vi "OAT Polar Plot Cursor Name on Picture.vi"(4 "avoid rect":T1(array[cluster]), 5 "[user-specified font]":T3, 6 "name above cursor":i32=5, 7 "desired font(Application)":T4(ring)=enum."Application Font", 8 "name":string, 9 "cursor position":cluster{"horizontal":i16, "vertical":i16}, 10 "cursor attributes":T5={"layout color"=852223, "active color"=16740820, "precision"=2, "BG transparent? (T)"=FALSE, "radius"=2}, 11 "picture":picture) -> (0 "text plotted":bool, 1 "text rect":T2, 3 "new picture":picture)   [LabVIEW 2017]
uses:
  <vilib>/addons/Sound and Vibration/Order Analysis/Backward Compatibility/SubVIs/OAT Polar Cursor Attributes.ctl
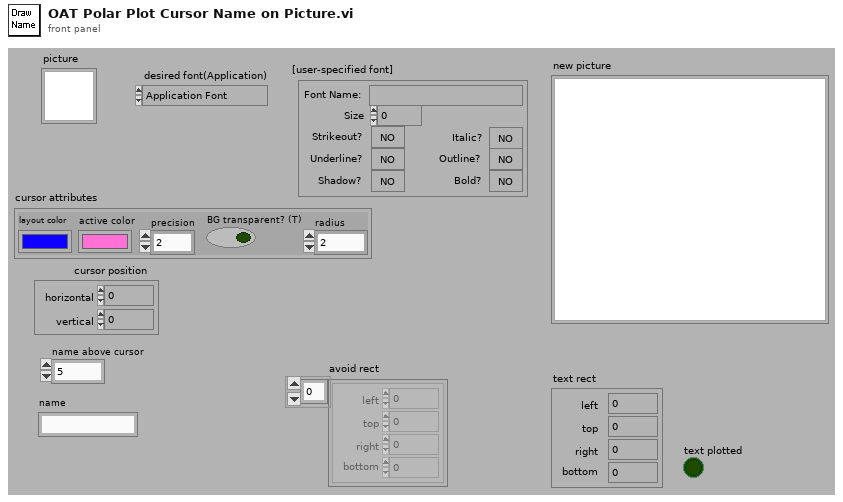
[diagram p1: front panel]
types:
  T1 = cluster{"left":i16, "top":i16, "right":i16, "bottom":i16}[]
  T2 = cluster{"left":i16, "top":i16, "right":i16, "bottom":i16}
  T3 = cluster{"Font Name:":string, "Size":i16, "Strikeout?":bool, "Italic?":bool, "Underline?":bool, "Outline?":bool, "Shadow?":bool, "Bold?":bool}
  T4 = enum16{"User-specified Font", "Application Font", "System Font", "Dialog Font"}
  T5 = typedef "OAT Polar Cursor Attributes.ctl" = cluster{"layout color":u32, "active color":u32, "precision":i16, "BG transparent? (T)":bool, "radius":i16}
  T6 = cluster{"horizontal":enum16{"left", "center", "right"}, "vertical":enum16{"top", "center", "bottom"}}
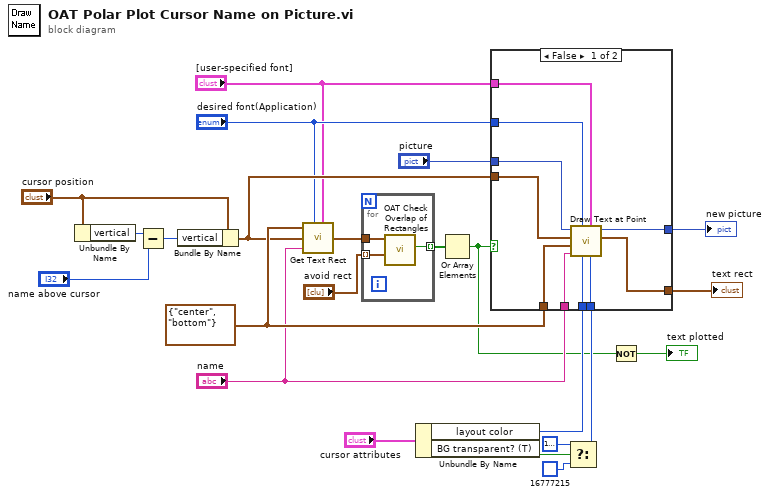
[diagram p0: block diagram]
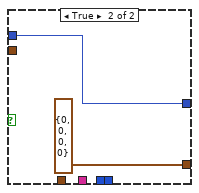
[diagram p2: hidden frame]
diagram:
  w10 = T6 {"horizontal"=enum."center", "vertical"=enum."bottom"} ("alignment(left, top)")
  n1 = Unbundle By Name("cursor position") -> ("vertical"=w22:i16)
  n2 = Subtract(x=w22, y="name above cursor") -> (x-y=w20:i32)
  n3 = Bundle By Name(cluster="cursor position", "vertical"=w20) -> (w9:cluster{"horizontal":i16, "vertical":i16})
  n4 = call <vilib>:"Get Text Rect.vi"("alignment(left, top)"=w10, "desired font(Application)"="desired font(Application)", "origin(0,0)"=w9, "text"="name", "[user-specified font]"="[user-specified font]") -> ("rect"=w5:T2)  [unwired: 4 in]
  n5 = for {
    tunnel: w5 -> [w26]
    tunnel: "avoid rect" -> [w25] mode=indexing
    tunnel: [w24] -> w3 mode=indexing
    n6 = call <vilib>:"OAT Check Overlap of Rectangles.vi"("rect 2"=w25, "rect 1"=w26) -> ("overlap"=w24:bool)  [unwired: 5 in]
  }
  n7 = Unbundle By Name("cursor attributes") -> ("layout color"=w15:u32, "BG transparent? (T)"=w14:bool)
  n8 = Or Array Elements(Boolean array=w3) -> (logical OR=w2:bool)
  n9 = Select(t=u32 16777216, s=w14, f=u32 16777215) -> (s? t:f=w17:u32)
  n10 = case shown="False" w2 {
    tunnel: "picture" -> [w36 w38]
    tunnel: w17 -> [w35 _]
    tunnel: [w34 w38] -> w16
    tunnel: w15 -> [w33 _]
    tunnel: [w32 T2 {"left"=0, "top"=0, "right"=0, "bottom"=0} ("text rect")] -> w11
    tunnel: w10 -> [w31 _]
    tunnel: w9 -> [w30 _]
    tunnel: "desired font(Application)" -> [w29 _]
    tunnel: "[user-specified font]" -> [w28 _]
    tunnel: "name" -> [w27 _]
    frame False {
      n11 = call <vilib>:"Draw Text at Point.vi"("BG color(transparent)"=w35, "[user-specified font]"=w28, "text color(black)"=w33, "desired font(Application)"=w29, "text"=w27, "alignment(left, top)"=w31, "origin"=w30, "picture"=w36) -> ("text rect"=w32:T2, "new picture"=w34:picture)  [unwired: 2 in]
    }
    frame True {
    }
  }
  "new picture" <- w16
  "text rect" <- w11
  n12 = Not(x=w2) -> (.not. x?=→"text plotted":bool)
